vi "Read GeneType.vi"(8 "error in":errorcluster, 11 "IGene in":refnum<class "IGene.lvclass">) -> (0 "error out":errorcluster, 2 "GeneType":T1, 3 "IGene out":refnum<class "IGene.lvclass">)   [LabVIEW 2016]
uses:
  _typedefs/IGene_GeneType.ctl
  IGene.lvclass
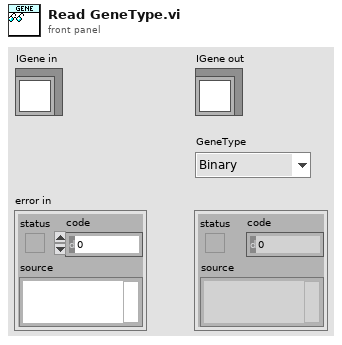
[diagram p1: front panel]
types:
  T1 = typedef "IGene.lvclass/IGene_GeneType.ctl" = enum16{"Binary", "Real", "Object", "None"}
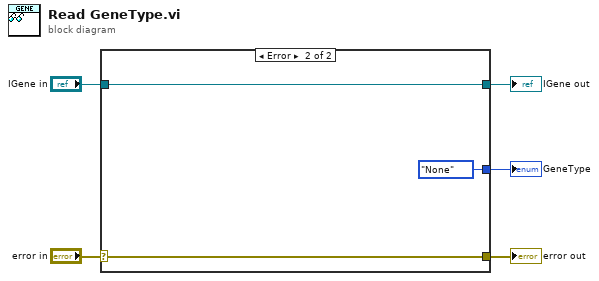
[diagram p0: block diagram]
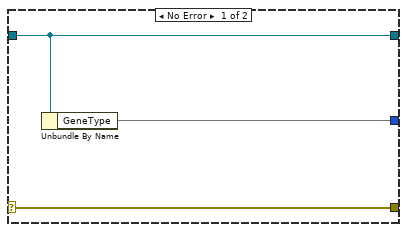
[diagram p2: hidden frame]
diagram:
  n1 = case shown="Error" "error in" {
    selector: "error in" -> [w8 w10]
    tunnel: [w8 w10] -> w4
    tunnel: [w7 w11] -> w2
    tunnel: "IGene in" -> [w7 w11]
    tunnel: [w6 IGene_GeneType."None" ("GeneType")] -> w1
    frame No Error {
      n2 = Unbundle By Name(w7) -> ("GeneType"=w6)
    }
    frame Error {
    }
  }
  "error out" <- w4
  "IGene out" <- w2
  "GeneType" <- w1
